vi "main.vi"() -> ()   [LabVIEW 2016]
uses:
  System Status.ctl
  Position Control.ctl
  Position Coordinate.ctl
  Manual Operation Control.ctl
panel:
  in  "MotionIni File In":path=path "C:/Program Files (x86)/National Instruments/LabVIEW 2016/user.lib/iselmotion/CNCAPI/CtrlDll/Dummy/MctlDummy.INI"
  in  "MotionLibrary Path":path=path "C:/Program Files (x86)/National Instruments/LabVIEW 2016/user.lib/iselmotion/CNCAPI/CtrlDll/Dummy/mctlDummy.dll"
  in  "Auto Run Control":T1[](array[typedef])
  in  "Auto Run":bool
  in  "Abs Position":T2={"Pos X"=0.0, "Position Name"="Abs Move", "Pos Y"=0.0, "Pos Z"=0.0, "Pos A"=0.0, "OK Button"=FALSE, "Normal Move"=FALSE, "Fast Move"=FALSE} {"Pos A" format="%.2f"; "Pos Z" format="%.2f"; "Pos Y" format="%.2f"; "Pos X" format="%.2f"}
  in  "Rel Position":T2={"Pos X"=0.0, "Position Name"="Rel Move", "Pos Y"=0.0, "Pos Z"=0.0, "Pos A"=0.0, "OK Button"=FALSE, "Normal Move"=FALSE, "Fast Move"=FALSE} {"Pos A" format="%.2f"; "Pos Z" format="%.2f"; "Pos Y" format="%.2f"; "Pos X" format="%.2f"}
  in  "Manual Operation Control":T3 {"Speed Override (%)" min=0.0 max=150.0 step=1.0 scale=0.0..150.0; "Rotative"."Step Length" min=0.01 max=100.0 step=0.01; "Rotative"."Speed" min=0.0 max=500.0 step=1.0 scale=0.0..500.0 scale format="%#.0f"; "Linear"."Step Length" min=0.01 max=500.0 step=0.01; "Linear"."Speed" min=0.0 max=500.0 step=1.0 scale=0.0..500.0 scale format="%#.0f"}
  out "Status":bool
  in  "Test Mode":bool
  in  "Leave HWLS":bool
  in  "Reference":bool
  in  "Reset Motion":bool
  in  "Stop Motion":bool
  in  "Settings":bool
  in  "Exit":bool
  in  "Initialize":bool
  out "System Status":T4 {"Axis A"."Position" format="%.2f"; "Axis Z"."Position" format="%.2f"; "Axis Y"."Position" format="%.2f"; "Rotativ Speed" format="%#_6f"; "Linear Speed" format="%#.2f"; "Axis X"."Position" format="%.2f"}
  out "Error Information":string
  out "Motor hModule":i32
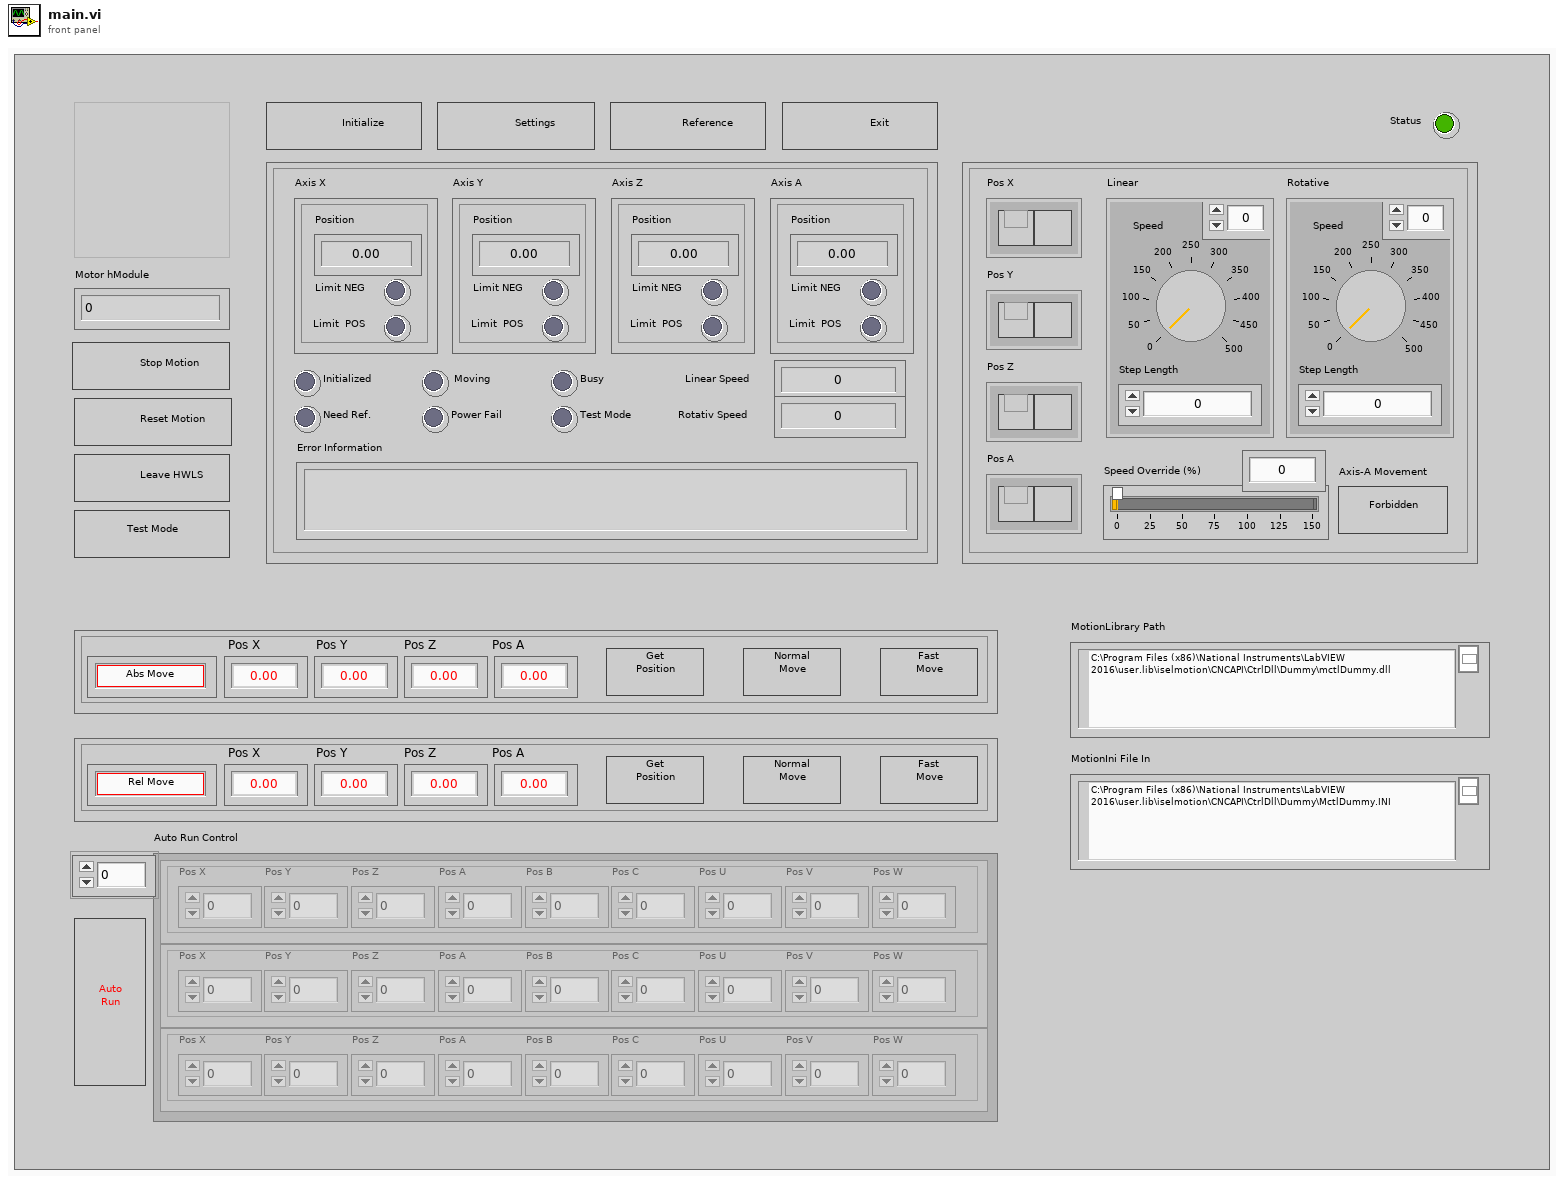
[diagram p1: front panel]
types:
  T1 = typedef "Position Coordinate.ctl" = cluster{"Pos X":dbl, "Pos Y":dbl, "Pos Z":dbl, "Pos A":dbl, "Pos B":dbl, "Pos C":dbl, "Pos U":dbl, "Pos V":dbl, "Pos W":dbl}
  T2 = typedef "Position Control.ctl" = cluster{"Pos X":dbl, "Position Name":string, "Pos Y":dbl, "Pos Z":dbl, "Pos A":dbl, "OK Button":bool, "Normal Move":bool, "Fast Move":bool}
  T3 = typedef "Manual Operation Control.ctl" = cluster{"Pos X":cluster{"Plus":bool, "Minus":bool}, "Pos Y":cluster{"Plus":bool, "Minus":bool}, "Pos Z":cluster{"Plus":bool, "Minus":bool}, "Pos A":cluster{"Plus":bool, "Minus":bool}, "Linear":cluster{"Speed":dbl, "Step Length":dbl}, "Rotative":cluster{"Speed":dbl, "Step Length":dbl}, "Speed Override (%)":dbl, "Axis-A Movement":bool}
  T4 = typedef "System Status.ctl" = cluster{"Axis X":cluster{"Position":dbl, "Limit NEG":bool, "Limit  POS":bool}, "Axis Y":cluster{"Position":dbl, "Limit NEG":bool, "Limit  POS":bool}, "Axis Z":cluster{"Position":dbl, "Limit NEG":bool, "Limit  POS":bool}, "Axis A":cluster{"Position":dbl, "Limit NEG":bool, "Limit  POS":bool}, "Initialized":bool, " Moving":bool, "Busy":bool, "Need Ref.":bool, "Power Fail":bool, "Test Mode":bool, "Linear Speed":dbl, "Rotativ Speed":dbl, "Error Information":string}
  T5 = enum16{"open", "replace", "create", "open or create", "replace or create", "replace or create with confirmation"}
  T6 = enum8{"Enabled", "Disabled", "Disabled and Grayed Out"}
  T7 = cluster{"PosX":i32, "PosY":i32, "PosZ":i32, "PosA":i32, "PosB":i32, "PosC":i32, "PosU":i32, "PosV":i32, "PosW":i32}
  T8 = cluster{"MotionLibrary Path":path, "MotionIni File In":path}
  T9 = cluster{"Common":cluster{"INMOTION":bool, "INSTOPMODE":bool, "INTEACHMODE":bool, "INTESTMODE":bool, "CURRENTOFF":bool, "INPATHMOTION":bool, "ISMOVING":bool, "PATHSTARTED":bool, "NEEDREFERENCERUN":bool, "BREAKERROR":bool, "HWLSACTIVE":bool, "SWLSACTIVE":bool, "HWLSDURINGMOTION":bool, "AFTERRUNERROR":bool, "LOADPATHDATAERROR":bool, "KEYSWITCHERROR":bool, "KEYSWDURINGMOTION":bool, "POWER_FAIL":bool, "SC_FAIL":bool, "HARDWARE_FAIL":bool, "COMMUNICATION_FAIL":bool}, "HWLSNeg":cluster{"HWLS_X_NEG":bool, "HWLS_Y_NEG":bool, "HWLS_Z_NEG":bool, "HWLS_A_NEG":bool, "HWLS_B_NEG":bool, "HWLS_C_NEG":bool, "HWLS_U_NEG":bool, "HWLS_V_NEG":bool, "HWLS_W_NEG":bool}, "HWLSPos":cluster{"HWLS_X_POS":bool, "HWLS_Y_POS":bool, "HWLS_Z_POS":bool, "HWLS_A_POS":bool, "HWLS_B_POS":bool, "HWLS_C_POS":bool, "HWLS_U_POS":bool, "HWLS_V_POS":bool, "HWLS_W_POS":bool}, "SWLSNeg":cluster{"SWLS_X_NEG":bool, "SWLS_Y_NEG":bool, "SWLS_Z_NEG":bool, "SWLS_A_NEG":bool, "SWLS_B_NEG":bool, "SWLS_C_NEG":bool, "SWLS_U_NEG":bool, "SWLS_V_NEG":bool, "SWLS_W_NEG":bool}, "SWLSPos":cluster{"SWLS_X_POS":bool, "SWLS_Y_POS":bool, "SWLS_Z_POS":bool, "SWLS_A_POS":bool, "SWLS_B_POS":bool, "SWLS_C_POS":bool, "SWLS_U_POS":bool, "SWLS_V_POS":bool, "SWLS_W_POS":bool}, "Extended":cluster{"ISBUSY":bool, "DISABLED":bool, "ISINITIALIZED":bool, "READY":bool, "DRILLCYCLEACTIVE":bool, "CTRLSPECERROR":bool}, "Additional flags":cluster{"InMotion":bool, "InStopMode":bool, "InTeachMode":bool, "InTestMode":bool, "CurrentOff":bool, "InPathMotion":bool, "IsMoving":bool, "NeedReferenceRun":bool, "BreakError":bool, "HWLSActive":bool, "SWLSActive":bool, "HWLSDuringMotion":bool, "AfterRunError":bool, "PowerFail":bool, "SCFail":bool, "IsBusy":bool, "Initialized":bool, "Disabled":bool, "HardwareFail":bool, "CommunicationFail":bool, "DrillCycleActive":bool, "CtrlSpecError":bool, "PathStarted":bool}}
  T10 = cluster{"PosX":dbl, "PosY":dbl, "PosZ":dbl, "PosA":dbl, "PosB":dbl, "PosC":dbl, "PosU":dbl, "PosV":dbl, "PosW":dbl}
  T11 = cluster{"PosX":dbl, "HWLS_X_NEG":bool, "HWLS_X_POS":bool}
  T12 = cluster{"PosY":dbl, "HWLS_Y_NEG":bool, "HWLS_Y_POS":bool}
  T13 = cluster{"PosZ":dbl, "HWLS_Z_NEG":bool, "HWLS_Z_POS":bool}
  T14 = cluster{dbl, "HWLS_A_NEG":bool, "HWLS_A_POS":bool}
  T15 = cluster{"LiNormVel":i32, "DrNormVel":i32, "LiFastVel":i32, "DrFastVel":i32, "LiTeachVel":i32, "DrTeachVel":i32, "LiActVel":i32, "DrActVel":i32}
  T16 = cluster{"LiNormVel":dbl, "DrNormVel":dbl, "LiFastVel":dbl, "DrFastVel":dbl, "LiTeachVel":dbl, "DrTeachVel":dbl, "LiActVel":dbl, "DrActVel":dbl}
  T17 = cluster{"Ability":cluster{"LINEAR":bool, "CIRCLE":bool, "HELIX":bool, "SPLINE":bool, "BEZIER":bool, "PRECALC":bool, "ONLINE":bool}, "NumAxis":u32, "AxisConfig":cluster{"AxisConfig 0":cluster{"Type":cluster{"LINEAR":bool, "ROT":bool}, "In Use":bool, "ID":u32, "RangeMin":u32, "RangeMax":u32}, "AxisConfig 1":cluster{"Type":cluster{"LINEAR":bool, "ROT":bool}, "In Use":bool, "ID":u32, "RangeMin":u32, "RangeMax":u32}, "AxisConfig 2":cluster{"Type":cluster{"LINEAR":bool, "ROT":bool}, "In Use":bool, "ID":u32, "RangeMin":u32, "RangeMax":u32}, "AxisConfig 3":cluster{"Type":cluster{"LINEAR":bool, "ROT":bool}, "In Use":bool, "ID":u32, "RangeMin":u32, "RangeMax":u32}, "AxisConfig 4":cluster{"Type":cluster{"LINEAR":bool, "ROT":bool}, "In Use":bool, "ID":u32, "RangeMin":u32, "RangeMax":u32}, "AxisConfig 5":cluster{"Type":cluster{"LINEAR":bool, "ROT":bool}, "In Use":bool, "ID":u32, "RangeMin":u32, "RangeMax":u32}, "AxisConfig 6":cluster{"Type":cluster{"LINEAR":bool, "ROT":bool}, "In Use":bool, "ID":u32, "RangeMin":u32, "RangeMax":u32}, "AxisConfig 7":cluster{"Type":cluster{"LINEAR":bool, "ROT":bool}, "In Use":bool, "ID":u32, "RangeMin":u32, "RangeMax":u32}, "AxisConfig 8":cluster{"Type":cluster{"LINEAR":bool, "ROT":bool}, "In Use":bool, "ID":u32, "RangeMin":u32, "RangeMax":u32}}}
  T18 = cluster{"In Use":bool, "In Use":bool, "In Use":bool, "In Use":bool, "In Use":bool, "In Use":bool, "In Use":bool, "In Use":bool, "In Use":bool}
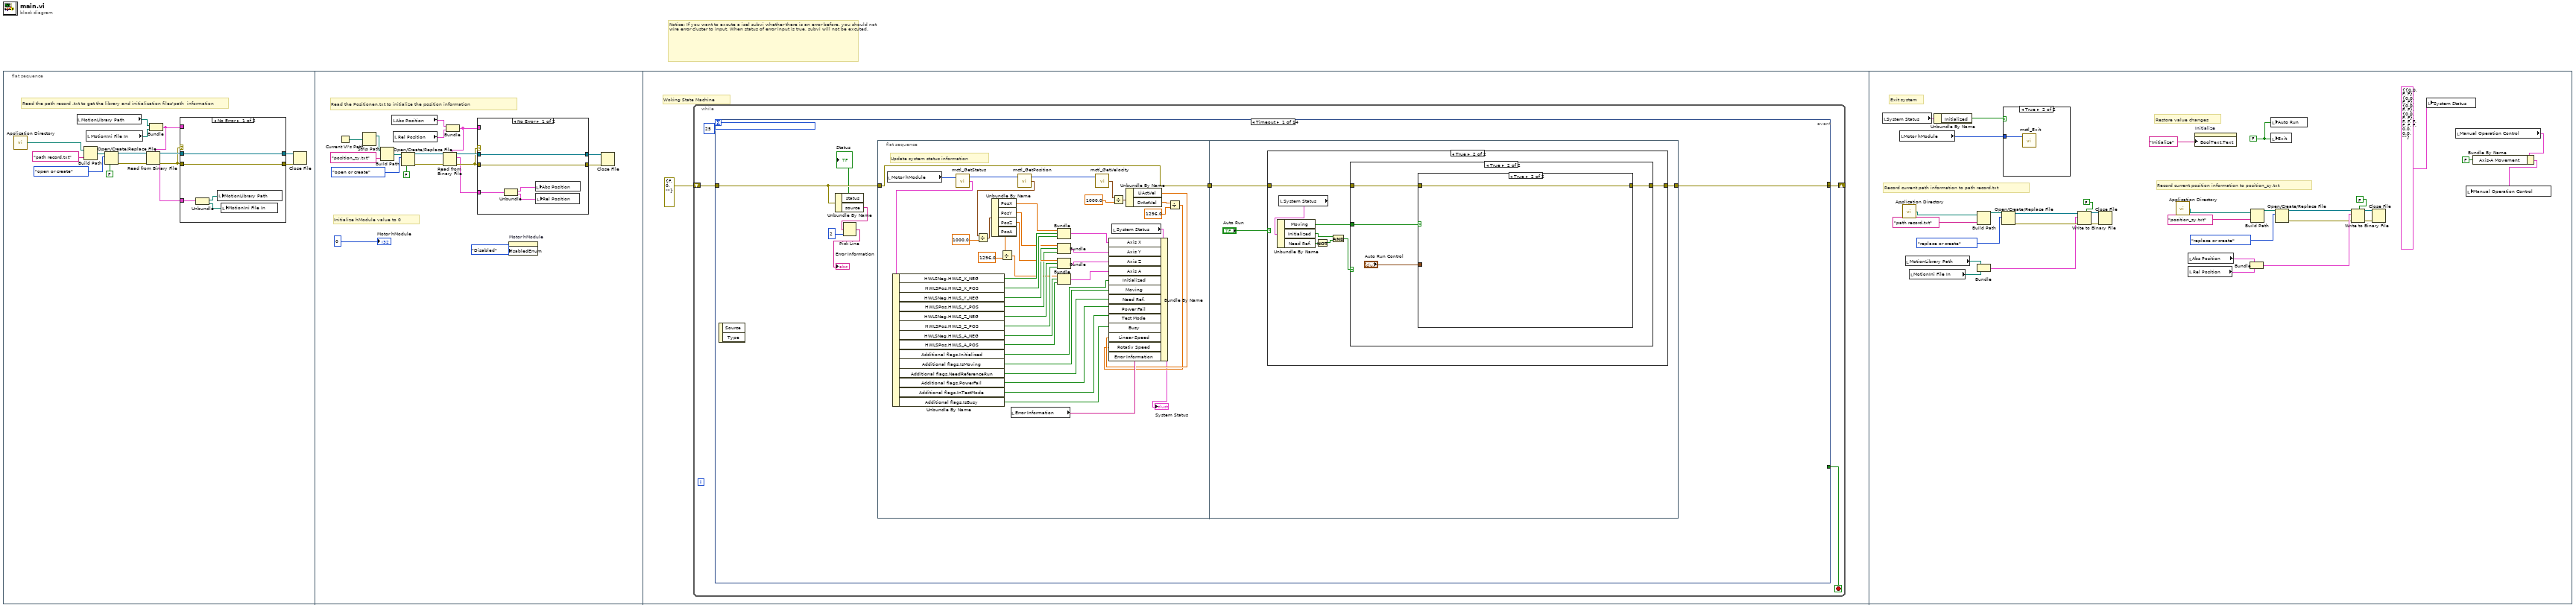
[diagram p0: block diagram]
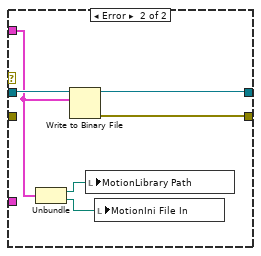
[diagram p2: hidden frame]
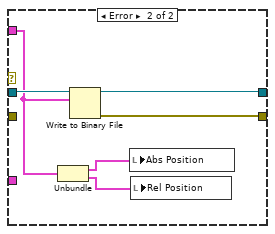
[diagram p3: hidden frame]
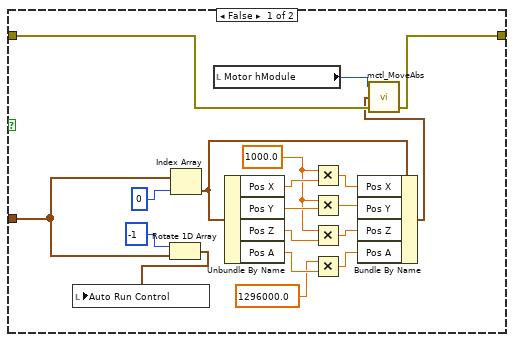
[diagram p6: hidden frame]
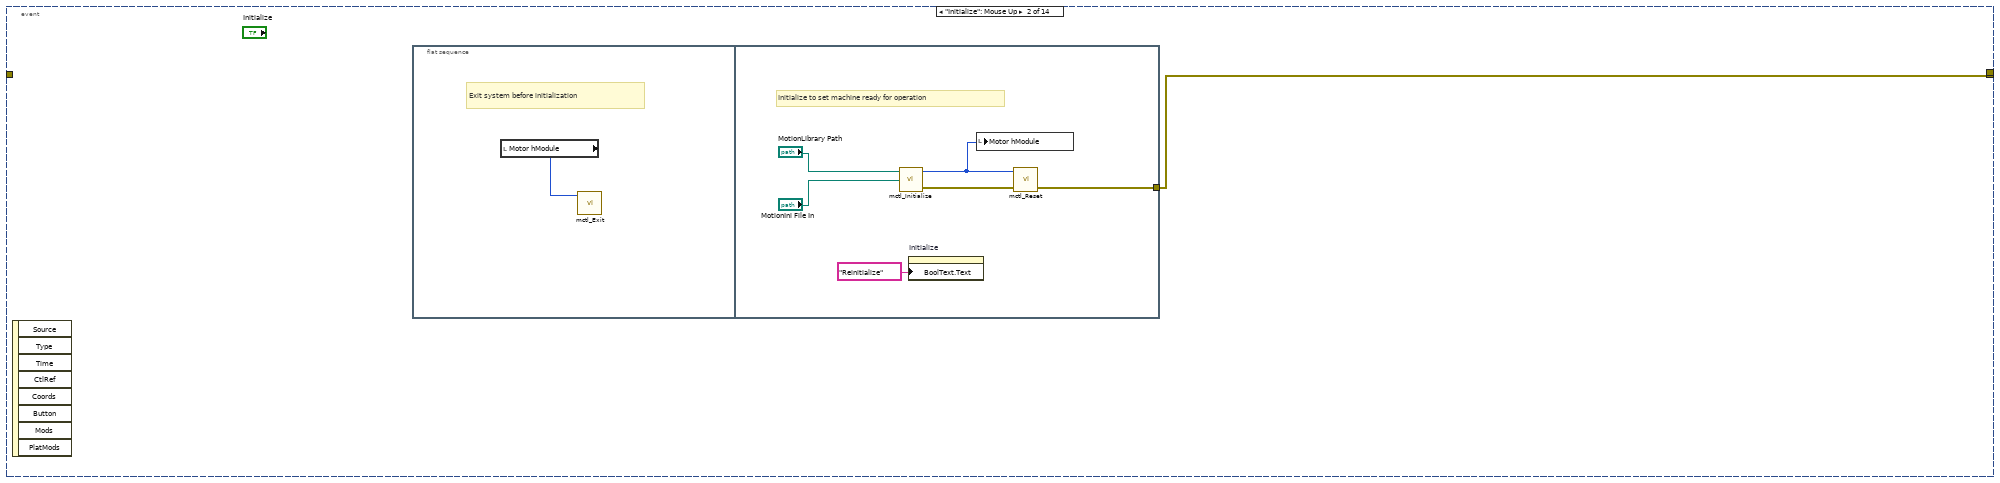
[diagram p7: hidden frame]
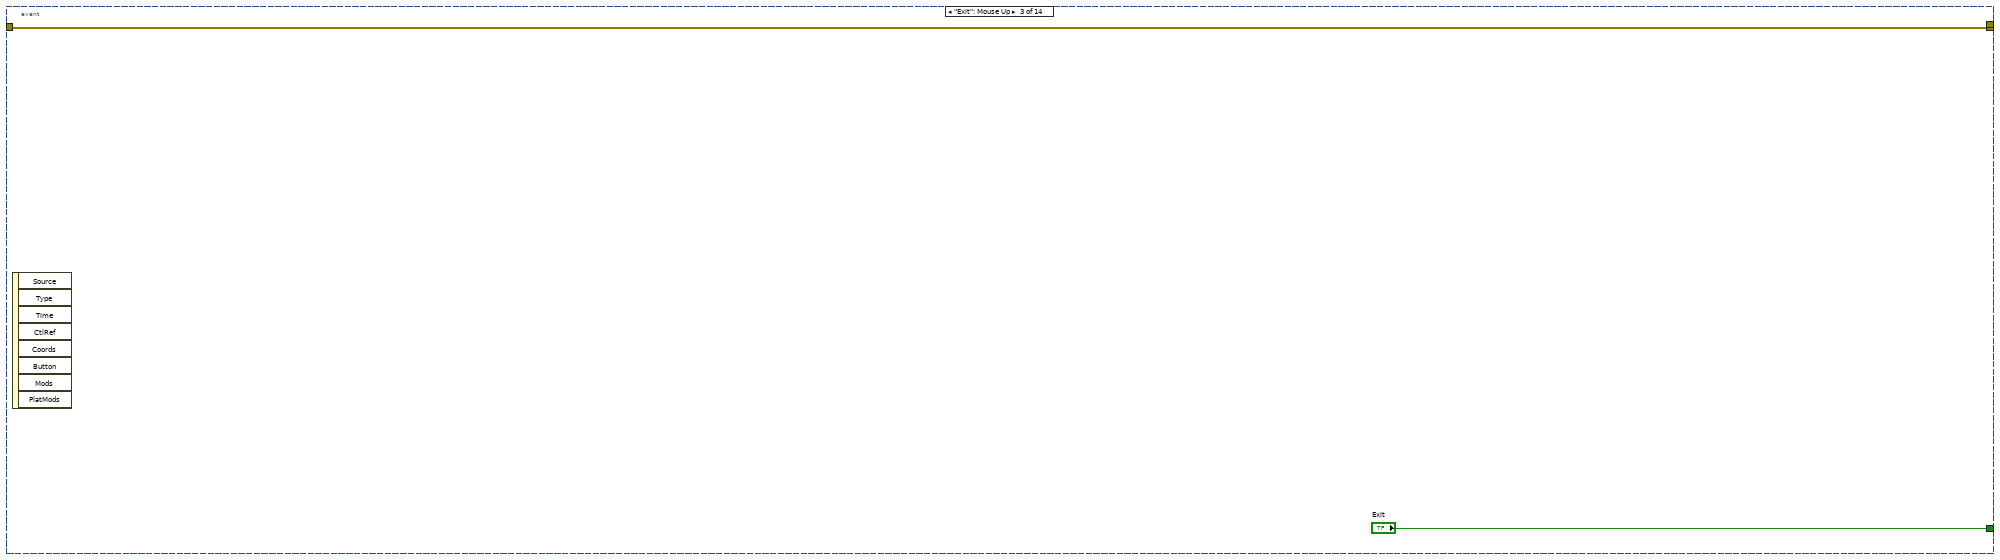
[diagram p8: hidden frame]
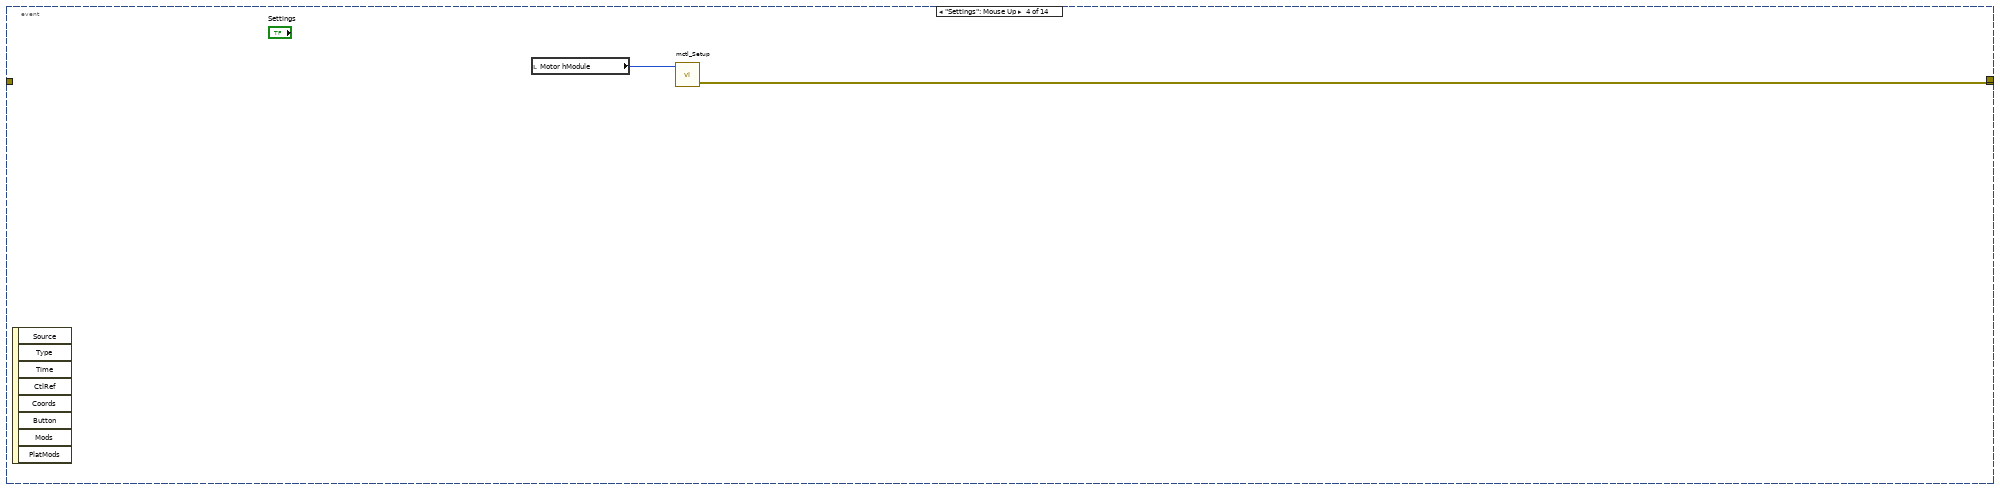
[diagram p9: hidden frame]
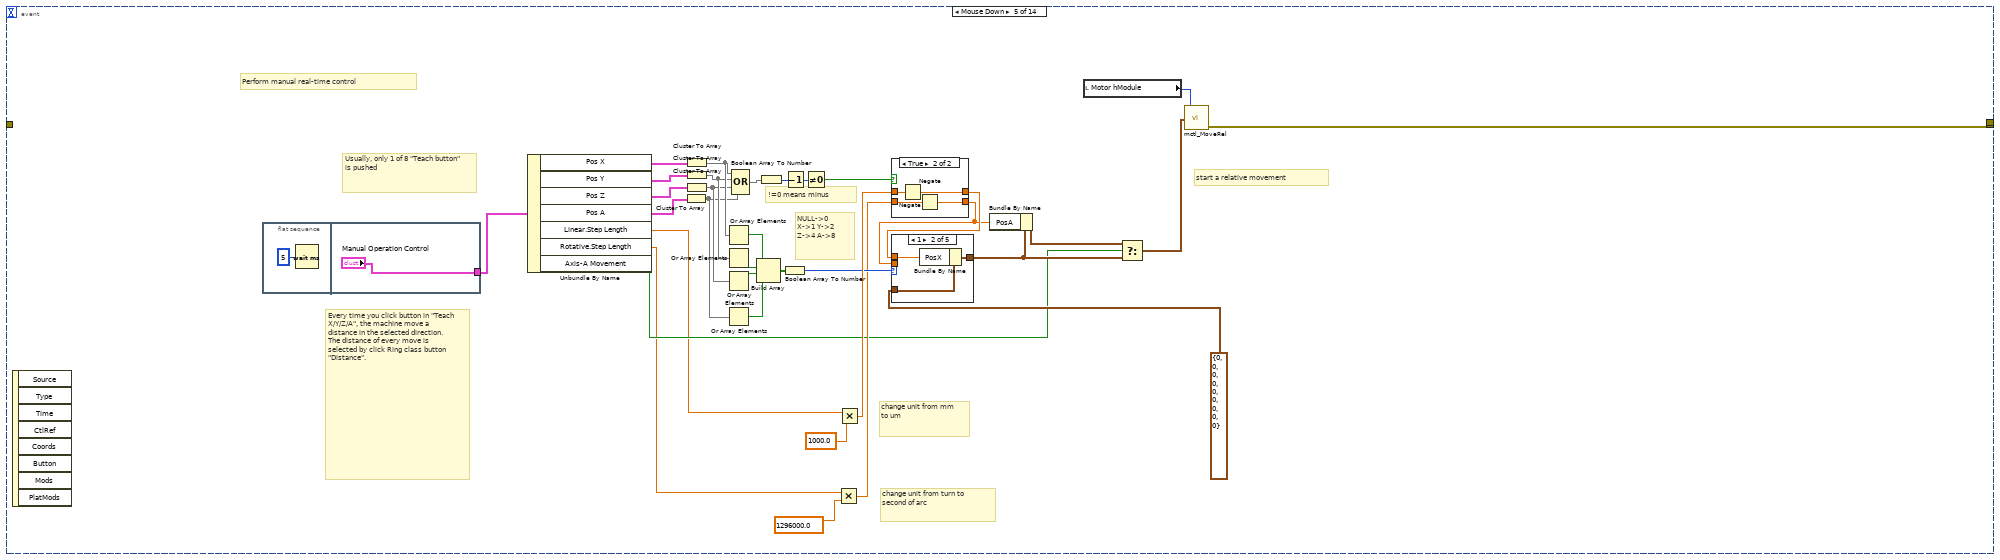
[diagram p10: hidden frame]
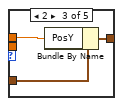
[diagram p12: hidden frame]
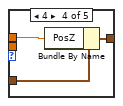
[diagram p13: hidden frame]
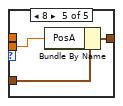
[diagram p14: hidden frame]
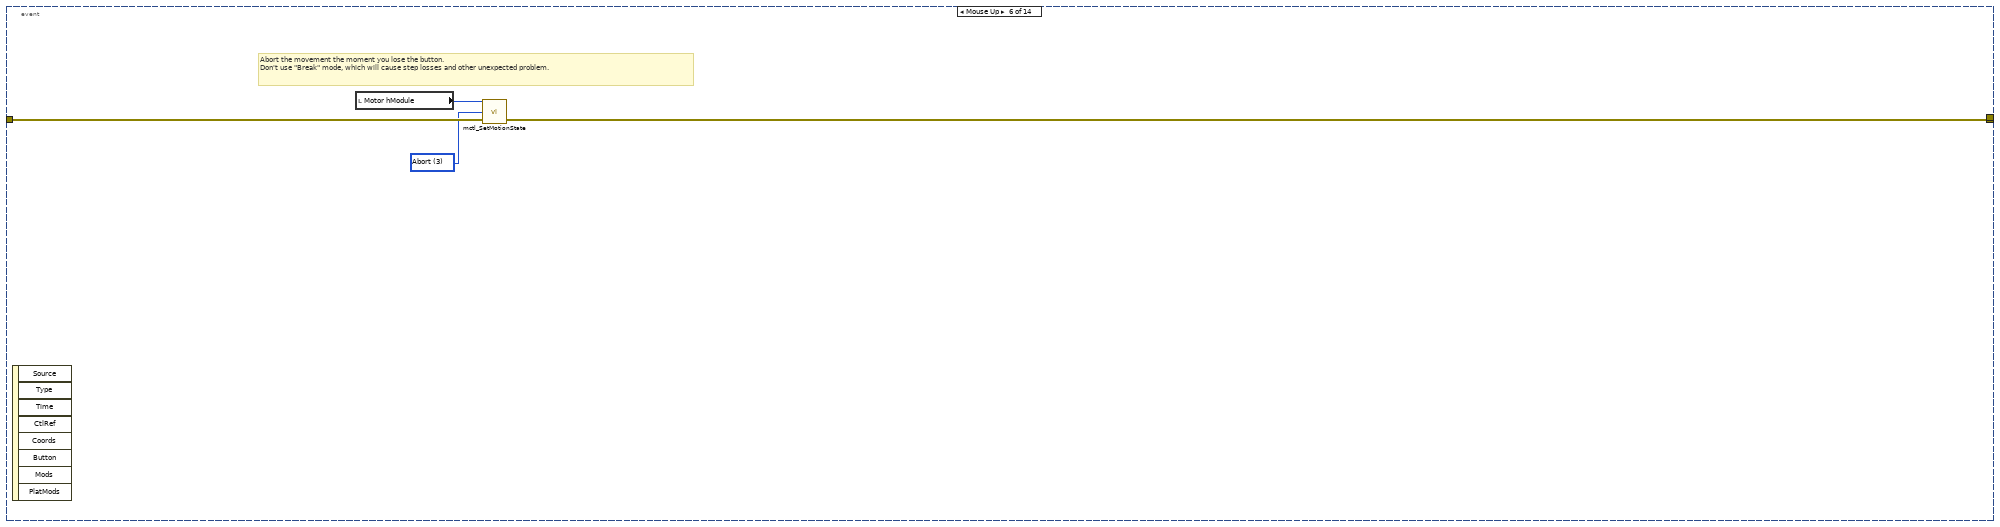
[diagram p16: hidden frame]
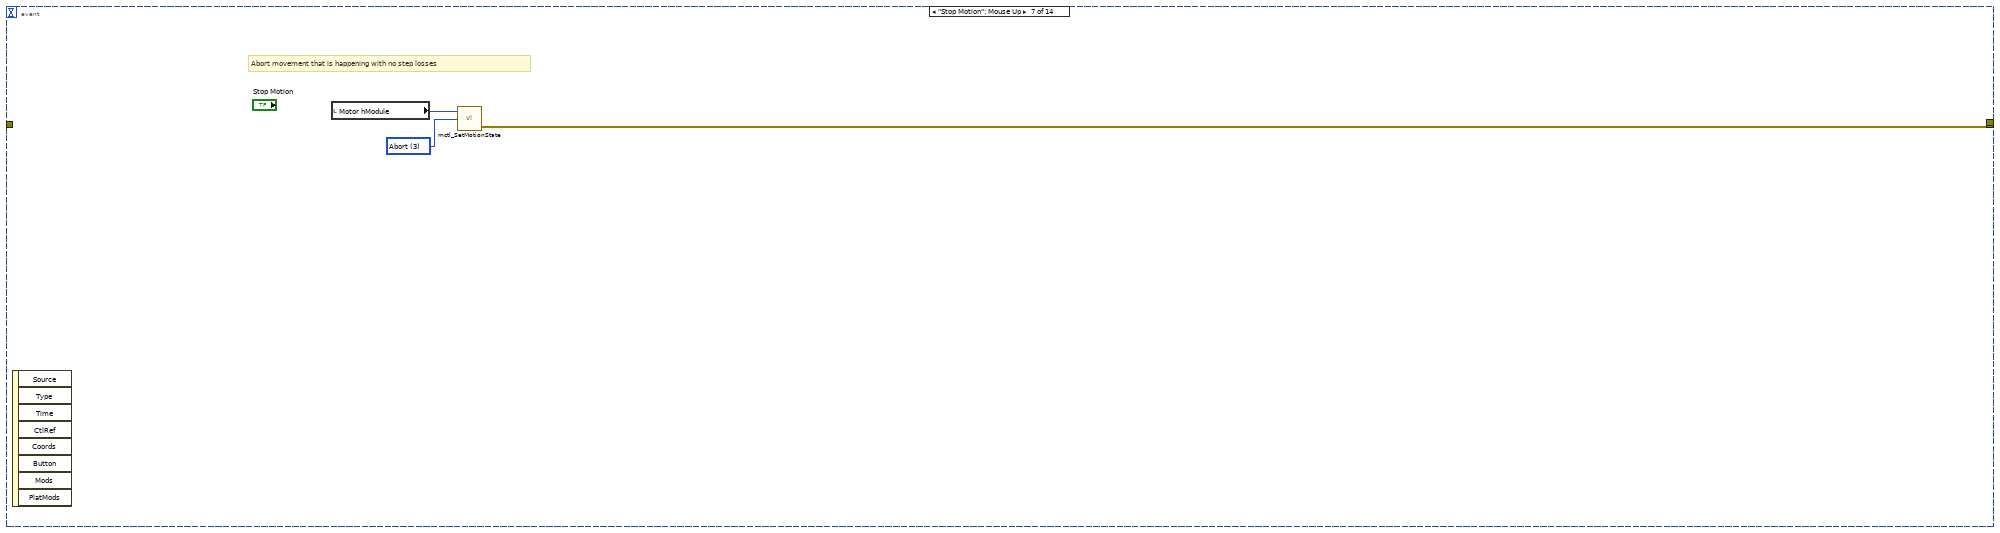
[diagram p17: hidden frame]
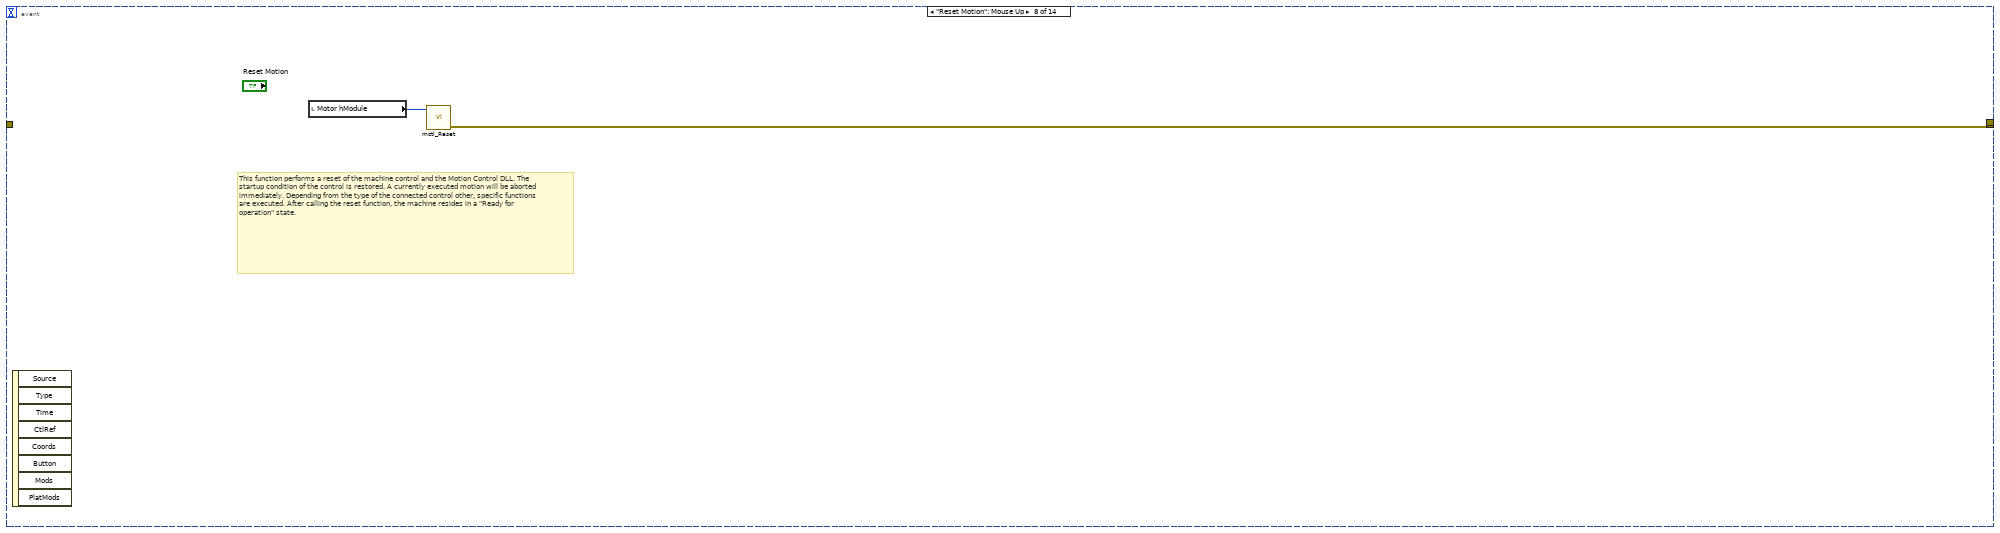
[diagram p18: hidden frame]
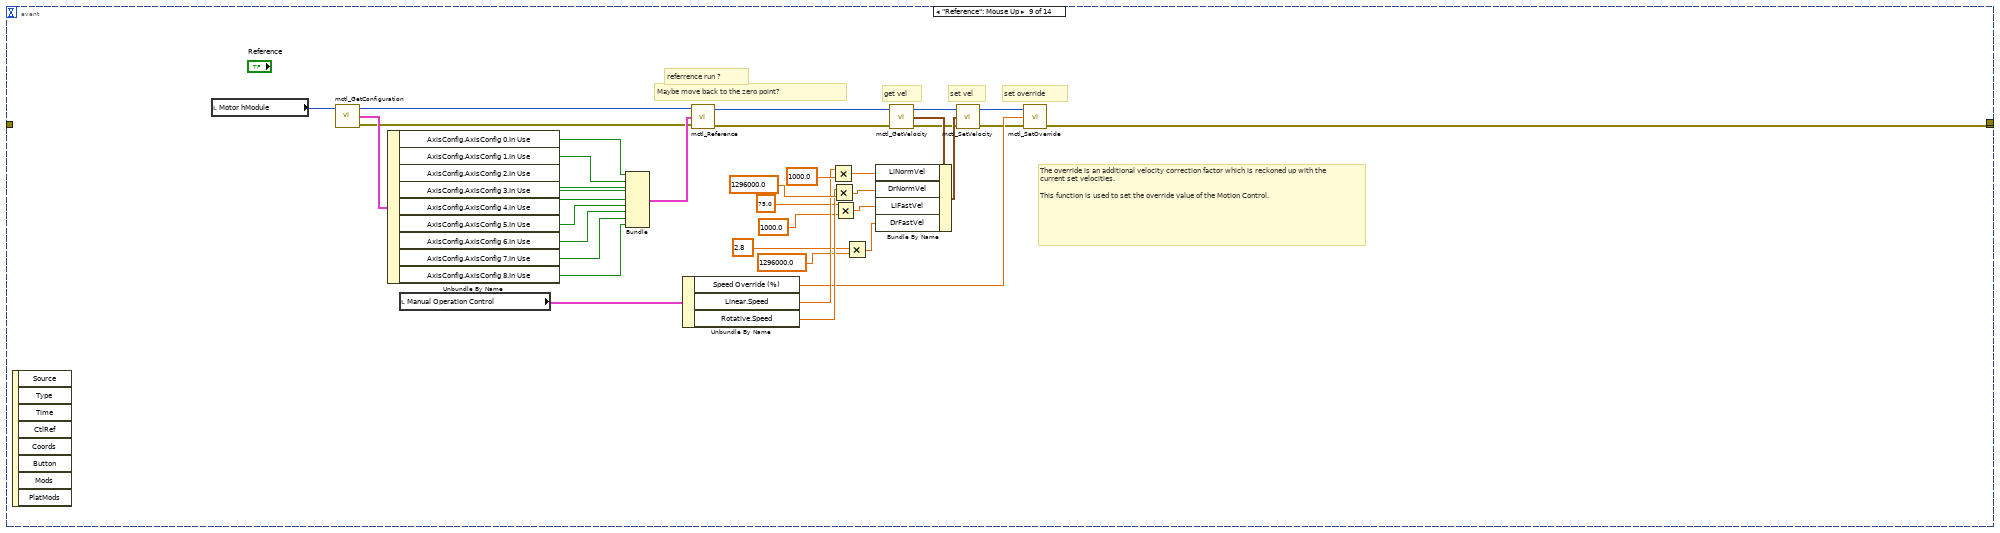
[diagram p19: hidden frame]
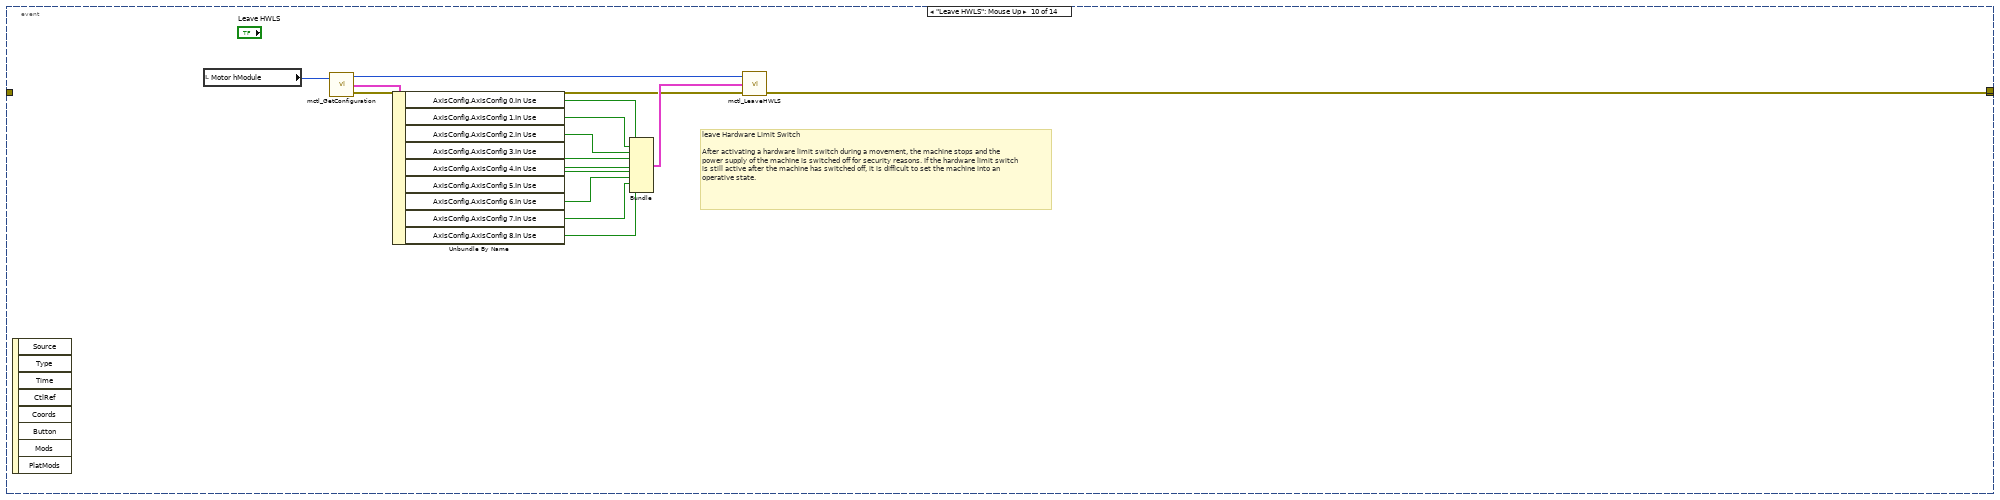
[diagram p20: hidden frame]
diagram:
  # "Notice: If you want to excute a isel subvi whether there is an error before, you should not wire error cluster to input. When status of error input is true, subvi will not be excuted."
  n1 = flat-sequence {
    frame #0 {
      # "Read the path record .txt to get the library and initialization files'path  information"
      n2 = call <vilib>:"Application Directory.vi"() -> ("Application Directory"=w2:path)
      n3 = local read "MotionLibrary Path"() -> (w10:path)
      n4 = Build Path(base path=w2, name or relative path="path record.txt") -> (appended path=w13:path)
      n5 = local read "MotionIni File In"() -> (w11:path)
      n6 = Open/Create/Replace File(file path (use dialog)=w13, operation (0:open)=T5."open or create", disable buffering (F)=FALSE ("advisory dialog? (display:T)")) -> (refnum out=w15:refnum<file>, error out=w12:errorcluster)  [unwired: 3 in, 1 out]
      n7 = Bundle("MotionLibrary Path"=w10, "MotionIni File In"=w11) -> (w3:T8)  [unwired: 1 in]
      n8 = Read from Binary File(5:w3, 8:w12, 11:w15) -> (0:w4:errorcluster, 2:w1:T8, 3:w7:refnum<file>)  [unwired: 3 in, 1 out]
      n9 = case shown="No Error" w4 {
        tunnel: w7 -> [w20 w26]
        tunnel: [w20 w24] -> w6
        tunnel: [w19 w25] -> w5
        tunnel: w4 -> [w19 _]
        tunnel: w3 -> [_ w23]
        tunnel: w1 -> [w18 _]
        frame No Error {
          n10 = Unbundle(w18) -> ("MotionLibrary Path"=w17:path, "MotionIni File In"=w16:path)
          n11 = local write "MotionLibrary Path"(w17) -> ()
          n12 = local write "MotionIni File In"(w16) -> ()
        }
        frame Error {
          n13 = Unbundle(w23) -> ("MotionLibrary Path"=w22:path, "MotionIni File In"=w21:path)
          n14 = Write to Binary File(file (use dialog)=w26, data=w23) -> (refnum out=w24:refnum<file>, error out=w25:errorcluster)  [unwired: 4 in, 1 out]
          n15 = local write "MotionLibrary Path"(w22) -> ()
          n16 = local write "MotionIni File In"(w21) -> ()
        }
      }
      n17 = Close File(refnum=w6, error in=w5) -> ()  [unwired: 2 out]
    }
    frame #1 {
      # "Initialize hModule value to 0"
      # "Read the Positionen.txt to initialize the position information"
      n18 = Current VI's Path() -> (path=w30:path)
      n19 = Strip Path(path=w30) -> (stripped path=w43:path)  [unwired: 1 out]
      n20 = Build Path(base path=w43, name or relative path="position_zy.txt") -> (appended path=w41:path)
      n21 = local read "Abs Position"() -> (w38:T2)
      n22 = local read "Rel Position"() -> (w39:T2)
      n23 = Open/Create/Replace File(file path (use dialog)=w41, operation (0:open)=T5."open or create", disable buffering (F)=FALSE ("advisory dialog? (display:T)")) -> (refnum out=w44:refnum<file>, error out=w40:errorcluster)  [unwired: 3 in, 1 out]
      n24 = Bundle("Abs Position"=w38, "Rel Position"=w39) -> (w31:cluster{"Abs Position":T2, "Rel Position":T2})  [unwired: 1 in]
      n25 = Read from Binary File(5:w31, 8:w40, 11:w44) -> (0:w32:errorcluster, 2:w28:cluster{"Abs Position":T2, "Rel Position":T2}, 3:w35:refnum<file>)  [unwired: 3 in, 1 out]
      n26 = case shown="No Error" w32 {
        tunnel: w35 -> [w49 w55]
        tunnel: [w49 w53] -> w34
        tunnel: [w48 w54] -> w33
        tunnel: w32 -> [w48 _]
        tunnel: w31 -> [_ w52]
        tunnel: w28 -> [w47 _]
        frame No Error {
          n27 = Unbundle(w47) -> ("Abs Position"=w46:T2, "Rel Position"=w45:T2)
          n28 = local write "Abs Position"(w46) -> ()
          n29 = local write "Rel Position"(w45) -> ()
        }
        frame Error {
          n30 = Unbundle(w52) -> ("Abs Position"=w51:T2, "Rel Position"=w50:T2)
          n31 = Write to Binary File(file (use dialog)=w55, data=w52) -> (refnum out=w53:refnum<file>, error out=w54:errorcluster)  [unwired: 4 in, 1 out]
          n32 = local write "Abs Position"(w51) -> ()
          n33 = local write "Rel Position"(w50) -> ()
        }
      }
      n34 = property on="Motor hModule" class="DigNum (strict)"("DisabledEnum"=T6."Disabled" ("Disabled")) -> ()  [unwired: 2 in, 2 out]
      n35 = Close File(refnum=w34, error in=w33) -> ()  [unwired: 2 out]
      "Motor hModule" <- 0
    }
    frame #2 {
      # "Woking State Machine"
      n36 = while {
        shift-right: [w58] -> _
        shift-left: errorcluster {"status"=FALSE, "code"=0, "source"=""} ("error constant") -> [w59]
        stop <- w57 stop-if-true
        n37 = event shown="[0] Timeout" {
          selector: _ -> [_ _ _ _ _ _ _ _ _ _ _ _ _ _]
          dyn-events: _ -> [_ _ _ _ _ _ _ _ _ _ _ _ _ _]
          timeout: 25 -> [_ _ _ _ _ _ _ _ _ _ _ _ _ _]
          tunnel: w59 -> [w67 _ w155 _ _ w217 _ _ _ _ _ w283 w333 _]
          tunnel: [w62 w147 w155 w157 w161 w216 w218 w221 w227 w266 w275 _ w332 w383] -> w58
          tunnel: [_ _ "Exit" _ _ _ _ _ _ _ _ _ _ _] -> w57
          tunnel: [_ _ _ _ _ _ _ _ _ _ _ w282 _ _] -> _
          event Timeout {
            n38 = event-data() -> ()  [unwired: 1 in, 2 out]
            n39 = Unbundle By Name(w67) -> ("status"=→"Status":bool, "source"=w65:string)
            n40 = Pick Line(multi-line string=w65, line index=2) -> (output string=→"Error Information":string)  [unwired: 1 in]
            n41 = flat-sequence {
              tunnel: w67 -> [w69]
              tunnel: [w69] -> w63
              tunnel: w63 -> [w111]
              tunnel: [w110] -> w62
              frame #0 {
                # "Update system status information"
                n42 = local read "Motor hModule"() -> (w109:i32)
                n43 = call <userlib>:"mctl_GetStatus.vi"("hModule In"=w109) -> ("Status"=w108:T9, "hModule Out"=w107:u32)  [unwired: 2 in, 1 out]
                n44 = Unbundle By Name(w108) -> ("HWLSNeg.HWLS_X_NEG"=w101:bool, "HWLSPos.HWLS_X_POS"=w100:bool, "HWLSNeg.HWLS_Y_NEG"=w97:bool, "HWLSPos.HWLS_Y_POS"=w96:bool, "HWLSNeg.HWLS_Z_NEG"=w95:bool, "HWLSPos.HWLS_Z_POS"=w94:bool, "HWLSNeg.HWLS_A_NEG"=w93:bool, "HWLSPos.HWLS_A_POS"=w92:bool, "Additional flags.Initialized"=w87:bool, "Additional flags.IsMoving"=w86:bool, "Additional flags.NeedReferenceRun"=w85:bool, "Additional flags.PowerFail"=w82:bool, "Additional flags.InTestMode"=w83:bool, "Additional flags.IsBusy"=w84:bool)
                n45 = local read "Error Information"() -> (w81:string)
                n46 = call <userlib>:"mctl_GetPosition.vi"("hModule In"=w107) -> ("AxisPos"=w105:T7, "hModule Out"=w106:u32)  [unwired: 2 in, 1 out]
                n47 = Divide(x=w105, y=1000.0) -> (x/y=w103:T10)
                n48 = Unbundle By Name(w103) -> ("PosX"=w102:dbl, "PosY"=w99:dbl, "PosZ"=w98:dbl, "PosA"=w79:dbl)
                n49 = Divide(x=w79, y=1296.0) -> (x/y=w77:dbl)
                n50 = Bundle("PosX"=w102, "HWLS_X_NEG"=w101, "HWLS_X_POS"=w100) -> (w91:T11)  [unwired: 1 in]
                n51 = Bundle("PosY"=w99, "HWLS_Y_NEG"=w97, "HWLS_Y_POS"=w96) -> (w90:T12)  [unwired: 1 in]
                n52 = Bundle("PosZ"=w98, "HWLS_Z_NEG"=w95, "HWLS_Z_POS"=w94) -> (w89:T13)  [unwired: 1 in]
                n53 = Bundle(w77, "HWLS_A_NEG"=w93, "HWLS_A_POS"=w92) -> (w88:T14)  [unwired: 1 in]
                n54 = call <userlib>:"mctl_GetVelocity.vi"("hModule In"=w106) -> ("Velocity"=w74:T15)  [unwired: 2 in, 2 out]
                n55 = Divide(x=w74, y=1000.0) -> (x/y=w75:T16)
                n56 = local read "System Status"() -> (w80:T4)
                n57 = Unbundle By Name(w75) -> ("LiActVel"=w76:dbl, "DrActVel"=w72:dbl)
                n58 = Divide(x=w72, y=1296.0) -> (x/y=w70:dbl)
                n59 = Bundle By Name(cluster=w80, "Axis X"=w91, "Axis Y"=w90, "Axis Z"=w89, "Axis A"=w88, "Initialized"=w87, "Moving"=w86, "Need Ref."=w85, "Power Fail"=w82, "Test Mode"=w83, "Busy"=w84, "Linear Speed"=w76, "Rotativ Speed"=w70, "Error Information"=w81) -> (→"System Status":T4)
              }
              frame #1 {
                n60 = case shown="True" "Auto Run" {
                  tunnel: w111 -> [w113 w120]
                  tunnel: [w113 w119] -> w110
                  frame False {
                  }
                  frame True {
                    n61 = local read "System Status"() -> (w121:T4)
                    n62 = Unbundle By Name(w121) -> ("Moving"=w118:bool, "Initialized"=w116:bool, "Need Ref."=w117:bool)
                    n63 = Not(x=w117) -> (.not. x?=w114:bool)
                    n64 = And(x=w116, y=w114) -> (x .and. y?=w115:bool)
                    n65 = case shown="True" w115 {
                      tunnel: w120 -> [w122 w126]
                      tunnel: [w122 w123] -> w119
                      tunnel: w118 -> [_ w124]
                      frame False {
                      }
                      frame True {
                        n66 = case shown="True" w124 {
                          tunnel: w126 -> [w143 w146]
                          tunnel: [w140 w146] -> w123
                          tunnel: "Auto Run Control" -> [w141 _]
                          frame False {
                            w134 = 1000.0
                            n67 = Rotate 1D Array(1:w141, 2:-1 ("n")) -> (0:w139:T1[])
                            n68 = local write "Auto Run Control"(w139) -> ()
                            n69 = Index Array(array=w141, index=0) -> (element=w132:T1)
                            n70 = local read "Motor hModule"() -> (w142:i32)
                            n71 = Unbundle By Name(w132) -> ("Pos X"=w138:dbl, "Pos Y"=w137:dbl, "Pos Z"=w136:dbl, "Pos A"=w135:dbl)
                            n72 = Multiply(x=w134, y=w138) -> (x*y=w131:dbl)
                            n73 = Multiply(x=w134, y=w137) -> (x*y=w130:dbl)
                            n74 = Multiply(x=w134, y=w136) -> (x*y=w129:dbl)
                            n75 = Multiply(x=1296000.0, y=w135) -> (x*y=w128:dbl)
                            n76 = Bundle By Name(cluster=w132, "Pos X"=w131, "Pos Y"=w130, "Pos Z"=w129, "Pos A"=w128) -> (w127:T1)
                            n77 = call <userlib>:"mctl_MoveAbs.vi"("error in"=w143, "Abs"=w127, "hModule In"=w142) -> ("error out"=w140:errorcluster)  [unwired: 1 in, 1 out]
                          }
                          frame True {
                          }
                        }
                      }
                    }
                  }
                }
              }
            }
          }
          event "Initialize": Mouse Up {
            n78 = event-data() -> ()  [unwired: 1 in, 8 out]
            n79 = flat-sequence {
              tunnel: [w153] -> w147
              frame #0 {
                # "Exit system before initialization"
                n80 = local read "Motor hModule"() -> (w148:i32)
                n81 = call <userlib>:"mctl_Exit.vi"("hModule In"=w148) -> ()  [unwired: 3 in, 2 out]
              }
              frame #1 {
                # "Initialize to set machine ready for operation"
                n82 = call <userlib>:"mctl_Initialize.vi"("Ini File In"="MotionIni File In", "Library In"="MotionLibrary Path") -> ("error out"=w154:errorcluster, "hModule Out"=w150:u32)  [unwired: 1 in, 1 out]
                n83 = property on="Initialize" class="Bool (strict)"("BoolText.Text"="Reinitialize" ("Boolean Text.Text")) -> ()  [unwired: 2 in, 2 out]
                n84 = local write "Motor hModule"(w150) -> ()
                n85 = call <userlib>:"mctl_Reset.vi"("error in"=w154, "hModule In"=w150) -> ("error out"=w153:errorcluster)  [unwired: 2 in, 1 out]
              }
            }
          }
          event "Exit": Mouse Up {
            n86 = event-data() -> ()  [unwired: 1 in, 8 out]
          }
          event "Settings": Mouse Up {
            n87 = event-data() -> ()  [unwired: 1 in, 8 out]
            n88 = local read "Motor hModule"() -> (w158:i32)
            n89 = call <userlib>:"mctl_Setup.vi"("hModule In"=w158) -> ("error out"=w157:errorcluster)  [unwired: 3 in, 1 out]
          }
          event Mouse Down {
            # "Usually, only 1 of 8 \"Teach button\" is pushed"
            # "!=0 means minus"
            # "change unit from turn to second of arc"
            # "change unit from mm to um"
            # "start a relative movement"
            # "Every time you click button in \"Teach X/Y/Z/A\", the machine move a distance in the selected direction. The distance of every move is selected by click Ring class button \"Distance\"."
            # "NULL->0\nX->1 Y->2\nZ->4 A->8"
            # "Perform manual real-time control"
            n90 = event-data() -> ()  [unwired: 1 in, 8 out]
            n91 = flat-sequence {
              tunnel: ["Manual Operation Control"] -> w164
              frame #0 {
                n92 = Wait (ms)(milliseconds to wait=u32 5) -> ()  [unwired: 1 out]
              }
              frame #1 {
              }
            }
            n93 = Unbundle By Name(w164) -> ("Pos X"=w192:cluster{"Plus":bool, "Minus":bool}, "Pos Y"=w191:cluster{"Plus":bool, "Minus":bool}, "Pos Z"=w190:cluster{"Plus":bool, "Minus":bool}, "Pos A"=w189:cluster{"Plus":bool, "Minus":bool}, "Linear.Step Length"=w160:dbl, "Rotative.Step Length"=w159:dbl, "Axis-A Movement"=w165:bool)
            n94 = Cluster To Array(cluster=w189) -> (array=w180:bool[])
            n95 = Cluster To Array(cluster=w192) -> (array=w183:bool[])
            n96 = Cluster To Array(cluster=w191) -> (array=w182:bool[])
            n97 = Cluster To Array(cluster=w190) -> (array=w181:bool[])
            n98 = Or Array Elements(Boolean array=w183) -> (logical OR=w188:bool)
            n99 = Or Array Elements(Boolean array=w182) -> (logical OR=w187:bool)
            n100 = Or Array Elements(Boolean array=w181) -> (logical OR=w186:bool)
            n101 = Or Array Elements(Boolean array=w180) -> (logical OR=w185:bool)
            n102 = Compound Arithmetic op=OR(w183, w182, w181, w180) -> (w177:bool[])
            n103 = Build Array(w188, w187, w186, w185) -> (w184:bool[])
            n104 = Boolean Array To Number(Boolean array=w177) -> (number=w179:u32)
            n105 = Boolean Array To Number(Boolean array=w184) -> (number=w174:u32)
            n106 = Decrement(x=w179) -> (x-1=w178:u32)
            n107 = Not Equal To 0?(x=w178) -> (x != 0?=w163:bool)
            n108 = Multiply(x=w159, y=1296000.0) -> (x*y=w170:dbl)
            n109 = Multiply(x=w160, y=1000.0) -> (x*y=w175:dbl)
            n110 = case shown="True" w163 {
              tunnel: w175 -> [w209 w213]
              tunnel: [w209 w212] -> w172
              tunnel: w170 -> [w208 w211]
              tunnel: [w208 w210] -> w168
              frame False {
              }
              frame True {
                n111 = Negate(x=w213) -> (-x=w212:dbl)
                n112 = Negate(x=w211) -> (-x=w210:dbl)
              }
            }
            n113 = case shown="1" w174 {
              tunnel: T7 {"PosX"=0, "PosY"=0, "PosZ"=0, "PosA"=0, "PosB"=0, "PosC"=0, "PosU"=0, "PosV"=0, "PosW"=0} ("RelPOS") -> [w195 w197 w200 w203 w206]
              tunnel: [w195 w198 w201 w204 w207] -> w169
              tunnel: w172 -> [_ w196 w199 w202 _]
              tunnel: w168 -> [_ _ _ _ w205]
              frame 0, Default {
              }
              frame 1 {
                n114 = Bundle By Name(cluster=w197, "PosX"=w196) -> (w198:T7)
              }
              frame 2 {
                n115 = Bundle By Name(cluster=w200, "PosY"=w199) -> (w201:T7)
              }
              frame 4 {
                n116 = Bundle By Name(cluster=w203, "PosZ"=w202) -> (w204:T7)
              }
              frame 8 {
                n117 = Bundle By Name(cluster=w206, "PosA"=w205) -> (w207:T7)
              }
            }
            n118 = Bundle By Name(cluster=w169, "PosA"=w168) -> (w167:T7)
            n119 = local read "Motor hModule"() -> (w162:i32)
            n120 = Select(t=w167, s=w165, f=w169) -> (s? t:f=w166:T7)
            n121 = call <userlib>:"mctl_MoveRel.vi"("RelPOS"=w166, "hModule In"=w162) -> ("error out"=w161:errorcluster)  [unwired: 2 in, 1 out]
          }
          event Mouse Up {
            w214 = u32 3 items=["Restart", "Stop", "Break", "Abort"] ("Motion State")
            # "Abort the movement the moment you lose the button.\nDon't use \"Break\" mode, which will cause step losses and other unexpected problem."
            n122 = event-data() -> ()  [unwired: 1 in, 8 out]
            n123 = local read "Motor hModule"() -> (w215:i32)
            n124 = call <userlib>:"mctl_SetMotionState.vi"("error in"=w217, "Motion State"=w214, "hModule In"=w215) -> ("error out"=w216:errorcluster)  [unwired: 1 in, 1 out]
          }
          event "Stop Motion": Mouse Up {
            w220 = u32 3 items=["Restart", "Stop", "Break", "Abort"] ("Motion State")
            # "Abort movement that is happening with no step losses"
            n125 = event-data() -> ()  [unwired: 1 in, 8 out]
            n126 = local read "Motor hModule"() -> (w219:i32)
            n127 = call <userlib>:"mctl_SetMotionState.vi"("Motion State"=w220, "hModule In"=w219) -> ("error out"=w218:errorcluster)  [unwired: 2 in, 1 out]
          }
          event "Reset Motion": Mouse Up {
            # "This function performs a reset of the machine control and the Motion Control DLL. The startup condition of the control is restored. A currently executed motion will be aborted immediately. Depending from the type of the connected control other, specific functions are executed. After calling the reset function, the machine resides in a \"Ready for operation\" state."
            n128 = event-data() -> ()  [unwired: 1 in, 8 out]
            n129 = local read "Motor hModule"() -> (w222:i32)
            n130 = call <userlib>:"mctl_Reset.vi"("hModule In"=w222) -> ("error out"=w221:errorcluster)  [unwired: 3 in, 1 out]
          }
          event "Reference": Mouse Up {
            # "The override is an additional velocity correction factor which is reckoned up with the current set velocities. \n\nThis function is used to set the override value of the Motion Control."
            # "Maybe move back to the zero point?"
            # "referrence run ?"
            # "set override"
            # "set vel"
            # "get vel"
            n131 = event-data() -> ()  [unwired: 1 in, 8 out]
            n132 = local read "Motor hModule"() -> (w232:i32)
            n133 = call <userlib>:"mctl_GetConfiguration.vi"("hModule In"=w232) -> ("error out"=w223:errorcluster, "Configuration"=w258:T17, "hModule Out"=w259:u32)  [unwired: 2 in]
            n134 = Unbundle By Name(w258) -> ("AxisConfig.AxisConfig 0.In Use"=w257:bool, "AxisConfig.AxisConfig 1.In Use"=w256:bool, "AxisConfig.AxisConfig 2.In Use"=w255:bool, "AxisConfig.AxisConfig 3.In Use"=w254:bool, "AxisConfig.AxisConfig 4.In Use"=w253:bool, "AxisConfig.AxisConfig 5.In Use"=w231:bool, "AxisConfig.AxisConfig 6.In Use"=w230:bool, "AxisConfig.AxisConfig 7.In Use"=w229:bool, "AxisConfig.AxisConfig 8.In Use"=w228:bool)
            n135 = local read "Manual Operation Control"() -> (w233:T3)
            n136 = Bundle("In Use"=w257, "In Use"=w256, "In Use"=w255, "In Use"=w254, "In Use"=w253, "In Use"=w231, "In Use"=w230, "In Use"=w229, "In Use"=w228) -> (w252:T18)  [unwired: 1 in]
            n137 = Unbundle By Name(w233) -> ("Speed Override (%)"=w238:dbl, "Linear.Speed"=w249:dbl, "Rotative.Speed"=w248:dbl)
            n138 = call <userlib>:"mctl_Reference.vi"("error in"=w223, "Reference Axis"=w252, "hModule In"=w259) -> ("error out"=w226:errorcluster, "hModule Out"=w237:u32)  [unwired: 1 in]
            n139 = Multiply(x=w249, y=1000.0) -> (x*y=w247:dbl)
            n140 = Multiply(x=w248, y=1296000.0) -> (x*y=w246:dbl)
            n141 = Multiply(x=75.0, y=1000.0) -> (x*y=w243:dbl)
            n142 = Multiply(x=2.8, y=1296000.0) -> (x*y=w242:dbl)
            n143 = call <userlib>:"mctl_GetVelocity.vi"("error in"=w226, "hModule In"=w237) -> ("error out"=w225:errorcluster, "Velocity"=w236:T15, "hModule Out"=w235:u32)  [unwired: 1 in]
            n144 = Bundle By Name(cluster=w236, "LiNormVel"=w247, "DrNormVel"=w246, "LiFastVel"=w243, "DrFastVel"=w242) -> (w239:T15)
            n145 = call <userlib>:"mctl_SetVelocity.vi"("error in"=w225, "Velocity"=w239, "hModule In"=w235) -> ("error out"=w224:errorcluster, "hModule Out"=w234:u32)  [unwired: 1 in]
            n146 = call <userlib>:"mctl_SetOverride.vi"("error in"=w224, "Override %"=w238, "hModule In"=w234) -> ("error out"=w227:errorcluster)  [unwired: 1 in, 1 out]
          }
          event "Leave HWLS": Mouse Up {
            # "leave Hardware Limit Switch \n\nAfter activating a hardware limit switch during a movement, the machine stops and the power supply of the machine is switched off for security reasons. If the hardware limit switch is still active after the machine has switched off, it is difficult to set the machine into an operative state."
            n147 = event-data() -> ()  [unwired: 1 in, 8 out]
            n148 = local read "Motor hModule"() -> (w267:i32)
            n149 = call <userlib>:"mctl_GetConfiguration.vi"("hModule In"=w267) -> ("error out"=w260:errorcluster, "Configuration"=w274:T17, "hModule Out"=w268:u32)  [unwired: 2 in]
            n150 = Unbundle By Name(w274) -> ("AxisConfig.AxisConfig 0.In Use"=w273:bool, "AxisConfig.AxisConfig 1.In Use"=w272:bool, "AxisConfig.AxisConfig 2.In Use"=w271:bool, "AxisConfig.AxisConfig 3.In Use"=w270:bool, "AxisConfig.AxisConfig 4.In Use"=w269:bool, "AxisConfig.AxisConfig 5.In Use"=w265:bool, "AxisConfig.AxisConfig 6.In Use"=w264:bool, "AxisConfig.AxisConfig 7.In Use"=w263:bool, "AxisConfig.AxisConfig 8.In Use"=w262:bool)
            n151 = Bundle("In Use"=w273, "In Use"=w272, "In Use"=w271, "In Use"=w270, "In Use"=w269, "In Use"=w265, "In Use"=w264, "In Use"=w263, "In Use"=w262) -> (w261:T18)  [unwired: 1 in]
            n152 = call <userlib>:"mctl_LeaveHWLS.vi"("error in"=w260, "Axis leave Limit"=w261, "hModule In"=w268) -> ("error out"=w266:errorcluster)  [unwired: 1 in, 1 out]
          }
          event "Test Mode": Mouse Up {
            # "Remarks \n\nNormally a Motion Control requires the execution of a reference run before it is fully operative. Since the reference run is not executed it is not possible to take access to the various movement functions of the Motion Control.\n \nIn some cases, e.g. during the start-up phase of working with a machine, it may be useful to access the movement functions without the previous execution of a reference run. The function mctl_SetTestMode() activates the so called \"Test mode\" which simulates a reference run if the complying function mctl_Reference() is called. //The current positions of each axis become the new machine zero point. //\n\nIn addition, the permanent checking of the hardware limit switches is switched off. The checking of hardware limit switches is used to set the Motion Control into an error state immediately after the activation of at least one hardware limit switch.// This feature enables you to move one or several axes into the mechanical stop for test purposes. //"
            n153 = event-data() -> ()  [unwired: 1 in, 8 out]
            n154 = local read "Motor hModule"() -> (w276:i32)
            n155 = call <userlib>:"mctl_GetStatus.vi"("hModule In"=w276) -> ("error out"=w277:errorcluster, "Status"=w281:T9, "hModule Out"=w278:u32)  [unwired: 2 in]
            n156 = Unbundle By Name(w281) -> ("Common.INTESTMODE"=w280:bool)
            n157 = Not(x=w280) -> (.not. x?=w279:bool)
            n158 = call <userlib>:"mctl_SetTestMode.vi"("error in"=w277, "Test Mode"=w279, "hModule In"=w278) -> ("error out"=w275:errorcluster)  [unwired: 1 in, 1 out]
          }
          event Mouse Down {
            n159 = event-data() -> ()  [unwired: 1 in, 8 out]
            n160 = flat-sequence {
              tunnel: ["Abs Position"] -> w285
              frame #0 {
                n161 = Wait (ms)(milliseconds to wait=u32 5) -> ()  [unwired: 1 out]
              }
              frame #1 {
              }
            }
            n162 = for {
              N: 1 -> [_]
              tunnel: w285 -> [w295]
              tunnel: [w308] -> w286
              tunnel: [w291] -> w282
              tunnel: w283 -> [w289]
              w302 = 1000
              n163 = Unbundle By Name(w295) -> ("OK Button"=w309:bool)
              n164 = Unbundle By Name(w295) -> ("Normal Move"=w292:bool, "Fast Move"=w294:bool, "Pos X"=w305:dbl, "Pos Y"=w304:dbl, "Pos Z"=w303:dbl, "Pos A"=w301:dbl)
              n165 = case shown="True" w309 {
                tunnel: w295 -> [w324 w330]
                tunnel: [w324 w325] -> w308
                frame False {
                }
                frame True {
                  n166 = local read "System Status"() -> (w331:T4)
                  n167 = Unbundle By Name(w331) -> ("Axis X.Position"=w329:dbl, "Axis Y.Position"=w328:dbl, "Axis Z.Position"=w327:dbl, "Axis A.Position"=w326:dbl)
                  n168 = Bundle By Name(cluster=w330, "Pos X"=w329, "Pos Y"=w328, "Pos Z"=w327, "Pos A"=w326) -> (w325:T2)
                }
              }
              n169 = local read "Motor hModule"() -> (w290:i32)
              n170 = Compound Arithmetic op=OR(w292, w294) -> (w293:bool)
              n171 = Multiply(x=w305, y=w302) -> (x*y=w299:dbl)
              n172 = Multiply(x=w304, y=w302) -> (x*y=w298:dbl)
              n173 = Multiply(x=w303, y=w302) -> (x*y=w297:dbl)
              n174 = Multiply(x=w301, y=1296000) -> (x*y=w296:dbl)
              n175 = Bundle By Name(cluster=T7 {"PosX"=0, "PosY"=0, "PosZ"=0, "PosA"=0, "PosB"=0, "PosC"=0, "PosU"=0, "PosV"=0, "PosW"=0} ("Abs"), "PosX"=w299, "PosY"=w298, "PosZ"=w297, "PosA"=w296) -> (w306:T7)
              n176 = case shown="True" w293 {
                tunnel: w306 -> [_ w315]
                tunnel: w292 -> [_ w314]
                tunnel: [w310 w313] -> w291
                tunnel: w290 -> [_ w312]
                tunnel: w289 -> [w310 w311]
                frame False {
                }
                frame True {
                  n177 = case shown="True" w314 {
                    tunnel: w315 -> [w319 w323]
                    tunnel: [w318 w322] -> w313
                    tunnel: w312 -> [w317 w321]
                    tunnel: w311 -> [w316 w320]
                    frame False {
                      n178 = call <userlib>:"mctl_FastAbs.vi"("error in"=w316, "FastAbs"=w319, "hModule In"=w317) -> ("error out"=w318:errorcluster)  [unwired: 1 in, 1 out]
                    }
                    frame True {
                      n179 = call <userlib>:"mctl_MoveAbs.vi"("error in"=w320, "Abs"=w323, "hModule In"=w321) -> ("error out"=w322:errorcluster)  [unwired: 1 in, 1 out]
                    }
                  }
                }
              }
            }
            n180 = local write "Abs Position"(w286) -> ()
          }
          event Mouse Down {
            n181 = event-data() -> ()  [unwired: 1 in, 8 out]
            n182 = flat-sequence {
              tunnel: ["Rel Position"] -> w335
              frame #0 {
                n183 = Wait (ms)(milliseconds to wait=u32 5) -> ()  [unwired: 1 out]
              }
              frame #1 {
              }
            }
            n184 = for {
              N: 1 -> [_]
              tunnel: w335 -> [w345]
              tunnel: [w358] -> w336
              tunnel: [w341] -> w332
              tunnel: w333 -> [w339]
              w352 = 1000
              n185 = Unbundle By Name(w345) -> ("OK Button"=w359:bool)
              n186 = Unbundle By Name(w345) -> ("Normal Move"=w342:bool, "Fast Move"=w344:bool, "Pos X"=w355:dbl, "Pos Y"=w354:dbl, "Pos Z"=w353:dbl, "Pos A"=w351:dbl)
              n187 = case shown="True" w359 {
                tunnel: w345 -> [w374 w380]
                tunnel: [w374 w375] -> w358
                frame False {
                }
                frame True {
                  n188 = local read "System Status"() -> (w381:T4)
                  n189 = Unbundle By Name(w381) -> ("Axis X.Position"=w379:dbl, "Axis Y.Position"=w378:dbl, "Axis Z.Position"=w377:dbl, "Axis A.Position"=w376:dbl)
                  n190 = Bundle By Name(cluster=w380, "Pos X"=w379, "Pos Y"=w378, "Pos Z"=w377, "Pos A"=w376) -> (w375:T2)
                }
              }
              n191 = local read "Motor hModule"() -> (w340:i32)
              n192 = Compound Arithmetic op=OR(w342, w344) -> (w343:bool)
              n193 = Multiply(x=w355, y=w352) -> (x*y=w349:dbl)
              n194 = Multiply(x=w354, y=w352) -> (x*y=w348:dbl)
              n195 = Multiply(x=w353, y=w352) -> (x*y=w347:dbl)
              n196 = Multiply(x=w351, y=1296000) -> (x*y=w346:dbl)
              n197 = Bundle By Name(cluster=T7 {"PosX"=0, "PosY"=0, "PosZ"=0, "PosA"=0, "PosB"=0, "PosC"=0, "PosU"=0, "PosV"=0, "PosW"=0} ("Abs"), "PosX"=w349, "PosY"=w348, "PosZ"=w347, "PosA"=w346) -> (w356:T7)
              n198 = case shown="True" w343 {
                tunnel: w356 -> [_ w365]
                tunnel: w342 -> [_ w364]
                tunnel: [w360 w363] -> w341
                tunnel: w340 -> [_ w362]
                tunnel: w339 -> [w360 w361]
                frame False {
                }
                frame True {
                  n199 = case shown="False" w364 {
                    tunnel: w365 -> [w369 w373]
                    tunnel: [w368 w372] -> w363
                    tunnel: w362 -> [w367 w371]
                    tunnel: w361 -> [w366 w370]
                    frame False {
                      n200 = call <userlib>:"mctl_FastRel.vi"("error in"=w366, "FastRel"=w369, "hModule In"=w367) -> ("error out"=w368:errorcluster)  [unwired: 1 in, 1 out]
                    }
                    frame True {
                      n201 = call <userlib>:"mctl_MoveRel.vi"("error in"=w370, "RelPOS"=w373, "hModule In"=w371) -> ("error out"=w372:errorcluster)  [unwired: 1 in, 1 out]
                    }
                  }
                }
              }
            }
            n202 = local write "Rel Position"(w336) -> ()
          }
          event Value Change {
            n203 = event-data() -> ()  [unwired: 1 in, 6 out]
            n204 = local read "Manual Operation Control"() -> (w384:T3)
            n205 = local read "Motor hModule"() -> (w382:i32)
            n206 = call <userlib>:"mctl_GetVelocity.vi"("hModule In"=w382) -> ("error out"=w389:errorcluster, "Velocity"=w388:T15, "hModule Out"=w390:u32)  [unwired: 2 in]
            n207 = Unbundle By Name(w384) -> ("Speed Override (%)"=w385:dbl, "Linear.Speed"=w395:dbl, "Rotative.Speed"=w394:dbl)
            n208 = Multiply(x=w395, y=1000.0) -> (x*y=w393:dbl)
            n209 = Multiply(x=w394, y=1296000.0) -> (x*y=w392:dbl)
            n210 = Bundle By Name(cluster=w388, "LiNormVel"=w393, "DrNormVel"=w392) -> (w391:T15)
            n211 = call <userlib>:"mctl_SetVelocity.vi"("error in"=w389, "Velocity"=w391, "hModule In"=w390) -> ("error out"=w386:errorcluster, "hModule Out"=w387:u32)  [unwired: 1 in]
            n212 = call <userlib>:"mctl_SetOverride.vi"("error in"=w386, "Override %"=w385, "hModule In"=w387) -> ("error out"=w383:errorcluster)  [unwired: 1 in, 1 out]
          }
        }
      }
    }
    frame #3 {
      w398 = FALSE ("Stop")
      # "Exit system"
      # "Restore value changes"
      # "Record current position information to position_zy.txt"
      # "Record current path information to path record.txt"
      n213 = local read "System Status"() -> (w403:T4)
      n214 = local read "Motor hModule"() -> (w404:i32)
      n215 = call <vilib>:"Application Directory.vi"() -> ("Application Directory"=w420:path)
      n216 = local read "MotionLibrary Path"() -> (w424:path)
      n217 = local read "MotionIni File In"() -> (w423:path)
      n218 = Unbundle By Name(w403) -> ("Initialized"=w402:bool)
      n219 = Bundle("MotionLibrary Path"=w424, "MotionIni File In"=w423) -> (w422:T8)  [unwired: 1 in]
      n220 = Build Path(base path=w420, name or relative path="path record.txt") -> (appended path=w429:path)
      n221 = Open/Create/Replace File(file path (use dialog)=w429, operation (0:open)=T5."replace or create") -> (refnum out=w428:refnum<file>, error out=w426:errorcluster)  [unwired: 4 in, 1 out]
      n222 = case shown="True" w402 {
        tunnel: w404 -> [_ w431]
        frame False {
        }
        frame True {
          n223 = call <userlib>:"mctl_Exit.vi"("hModule In"=w431) -> ()  [unwired: 3 in, 2 out]
        }
      }
      n224 = Write to Binary File(file (use dialog)=w428, data=w422, error in=w426, 5:FALSE ("prepend array or string size? (T)")) -> (refnum out=w427:refnum<file>, error out=w425:errorcluster)  [unwired: 2 in, 1 out]
      n225 = Close File(refnum=w427, error in=w425) -> ()  [unwired: 2 out]
      n226 = call <vilib>:"Application Directory.vi"() -> ("Application Directory"=w417:path)
      n227 = local read "Abs Position"() -> (w413:T2)
      n228 = local read "Rel Position"() -> (w414:T2)
      n229 = property on="Initialize" class="Bool (strict)"("BoolText.Text"="Initialize" ("Boolean Text.Text")) -> ()  [unwired: 2 in, 2 out]
      n230 = Bundle("Abs Position"=w413, "Rel Position"=w414) -> (w415:cluster{"Abs Position":T2, "Rel Position":T2})  [unwired: 1 in]
      n231 = Build Path(base path=w417, name or relative path="position_zy.txt") -> (appended path=w408:path)
      n232 = local write "Auto Run"(w398) -> ()
      n233 = local write "Exit"(w398) -> ()
      n234 = Open/Create/Replace File(file path (use dialog)=w408, operation (0:open)=T5."replace or create") -> (refnum out=w409:refnum<file>, error out=w411:errorcluster)  [unwired: 4 in, 1 out]
      n235 = Write to Binary File(file (use dialog)=w409, data=w415, error in=w411, 5:FALSE ("prepend array or string size? (T)")) -> (refnum out=w410:refnum<file>, error out=w412:errorcluster)  [unwired: 2 in, 1 out]
      n236 = Close File(refnum=w410, error in=w412) -> ()  [unwired: 2 out]
      n237 = local write "System Status"(T4 {"Axis X"={"Position"=0.0, "Limit NEG"=FALSE, "Limit  POS"=FALSE}, "Axis Y"={"Position"=0.0, "Limit NEG"=FALSE, "Limit  POS"=FALSE}, "Axis Z"={"Position"=0.0, "Limit NEG"=FALSE, "Limit  POS"=FALSE}, "Axis A"={"Position"=0.0, "Limit NEG"=FALSE, "Limit  POS"=FALSE}, "Initialized"=FALSE, " Moving"=FALSE, "Busy"=FALSE, "Need Ref."=FALSE, "Power Fail"=FALSE, "Test Mode"=FALSE, "Linear Speed"=0.0, "Rotativ Speed"=0.0, "Error Information"=""} ("System Status")) -> ()
      n238 = local read "Manual Operation Control"() -> (w401:T3)
      n239 = Bundle By Name(cluster=w401, "Axis-A Movement"=FALSE) -> (w399:T3)
      n240 = local write "Manual Operation Control"(w399) -> ()
    }
  }
